vi "SmartSort.vi"(11 "Array in":cluster{"Numeric":i32, "Slide":dbl}[](array[cluster])) -> (3 "Array out":cluster{"Numeric":i32, "Slide":dbl}[](array[cluster]))   [LabVIEW 2016]
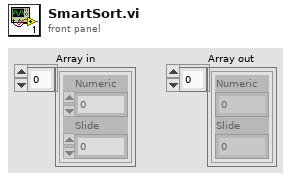
[diagram p1: front panel]
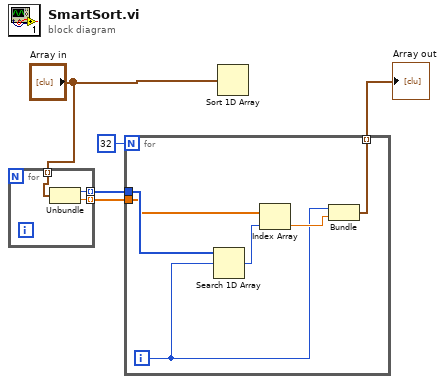
[diagram p0: block diagram]
diagram:
  n1 = for {
    tunnel: "Array in" -> [w8] mode=indexing
    tunnel: [w7] -> w3 mode=indexing
    tunnel: [w6] -> w2 mode=indexing
    n2 = Unbundle(w8) -> ("Numeric"=w7:i32, "Slide"=w6:dbl)
  }
  n3 = for {
    N: 32 -> [_]
    tunnel: w3 -> [w14]
    tunnel: w2 -> [w12]
    tunnel: [w9] -> w1 mode=indexing
    i -> [w10]
    n4 = Search 1D Array(1D array=w14, element=w10) -> (index of element=w13:i32)  [unwired: 1 in]
    n5 = Index Array(array=w12, index=w13) -> (element=w11:dbl)
    n6 = Bundle(w10, "Slide"=w11) -> (w9:cluster{i32, "Slide":dbl})  [unwired: 1 in]
  }
  "Array out" <- w1
  n7 = Sort 1D Array(array="Array in") -> ()  [unwired: 1 out]
